vi "Multi Recorder Query.vi"(0 "System no.":i32=1 min=1 max=4 step=1, 1 "Recorder Command":string, 2 "RecorderIDs to query":string[](array[string]), 5 "error in":errorcluster) -> (14 "Answer":string, 19 "error out":errorcluster)   [LabVIEW 2020]
doc: "Query multiple recorder infos."
panel:
  # "Query multiple recorder infos."
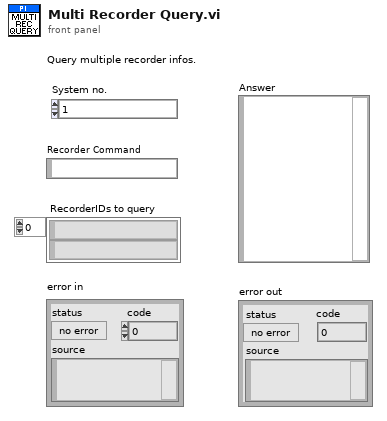
[diagram p1: front panel]
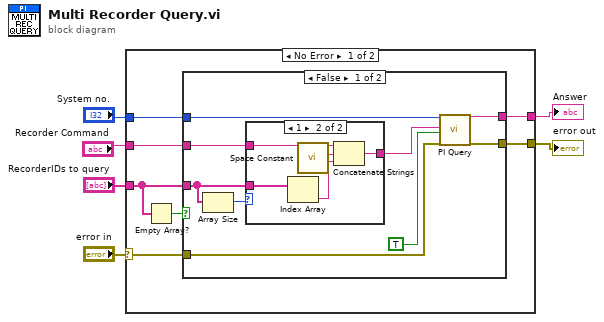
[diagram p0: block diagram]
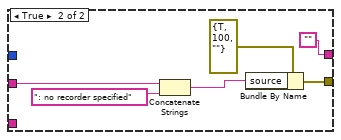
[diagram p3: hidden frame]
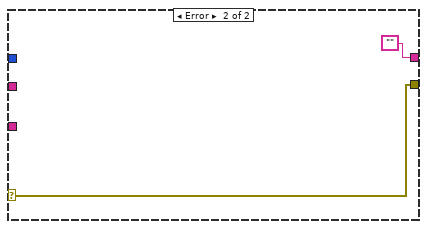
[diagram p4: hidden frame]
diagram:
  n1 = case shown="No Error" "error in" {
    selector: "error in" -> [w10 w36]
    tunnel: [w13 "" ("String read")] -> w6
    tunnel: "RecorderIDs to query" -> [w7 _]
    tunnel: [w12 w36] -> w5
    tunnel: "Recorder Command" -> [w11 _]
    tunnel: "System no." -> [w9 _]
    frame No Error {
      n2 = Empty Array?(array=w7) -> (empty?=w8:bool)
      n3 = case shown="False" w8 {
        tunnel: w9 -> [w20 _]
        tunnel: w7 -> [w14 _]
        tunnel: w10 -> [w16 _]
        tunnel: [w17 w33] -> w12
        tunnel: w11 -> [w19 w30]
        tunnel: [w18 "" ("String read")] -> w13
        frame False {
          n4 = Array Size(array=w14) -> (size(s)=w15:i32)
          n5 = case shown="1" w15 {
            tunnel: [w23 w28] -> w21
            tunnel: w14 -> [_ w27]
            tunnel: w19 -> [w23 w26]
            frame 0, Default {
            }
            frame 1 {
              n6 = Index Array(array=w27) -> (element=w25:string)  [unwired: 1 in]
              n7 = call <vilib>:"Space Constant.vi"() -> ("String"=w24:string)
              n8 = Concatenate Strings(w26, w24, w25) -> (w28:string)
            }
          }
          n9 = call "PI Query.vi"("System no."=w20, "String to send"=w21, "Attach termination char.?"=TRUE ("Attach Linefeed?"), "error in"=w16) -> ("String read"=w18:string, "error out"=w17:errorcluster)  [unwired: 3 in, 11 out]
        }
        frame True {
          n10 = Concatenate Strings(w30, ": no recorder specified" ("source")) -> (w32:string)
          n11 = Bundle By Name(cluster=errorcluster {"status"=TRUE, "code"=100, "source"=""} ("error out"), "source"=w32) -> (w33:errorcluster)
        }
      }
    }
    frame Error {
    }
  }
  "error out" <- w5
  "Answer" <- w6
